vi "Enable SPI Digital Lines(CLIP).vi"(7 "Set?":bool=TRUE, 8 "error in":errorcluster, 9 "Enable":bool[](array[boolean])=[TRUE, FALSE, TRUE, TRUE, TRUE, TRUE, TRUE, TRUE, TRUE], 10 "Enable Lines":T1={"SCLK_en"="sbRIO-9651 Socket\\PMOD1_Pin3_enable", "MISO_en"="sbRIO-9651 Socket\\PMOD1_Pin3_enable", "MOSI_en"="sbRIO-9651 Socket\\PMOD1_Pin3_enable", "CS0_en"="sbRIO-9651 Socket\\PMOD1_Pin3_enable", "CS1_en"="sbRIO-9651 Socket\\PMOD1_Pin3_enable", "CS2_en"="sbRIO-9651 Socket\\PMOD1_Pin3_enable", "CS3_en"="sbRIO-9651 Socket\\PMOD1_Pin3_enable", "CS4_en"="sbRIO-9651 Socket\\PMOD1_Pin3_enable", "CS5_en"="sbRIO-9651 Socket\\PMOD1_Pin3_enable"}, 11 "SPI DIO Lines":T2={"SCLK"="Port0/DIO0", "MISO"="Port0/DIO1", "MOSI"="Port0/DIO2", "CS 0"="Port0/DIO4", "CS 1"="Port0/DIO5", "CS 2"="Port0/DIO6", "CS 3"="Port0/DIO7", "CS 4"="Port0/DIO8", "CS 5"="Port0/DIO9"}) -> (0 "error out":errorcluster, 3 "Chip Select DIO Lines":T2={"SCLK"="Port0/DIO3", "MISO"="Port0/DIO3", "MOSI"="Port0/DIO3", "CS 0"="Port0/DIO4", "CS 1"="Port0/DIO4", "CS 2"="Port0/DIO1", "CS 3"="Port0/DIO4", "CS 4"="Port0/DIO4", "CS 5"="Port0/DIO4"})   [LabVIEW 2014]
uses:
  <vilib>/SPIAPI/DIO/SPI Digital IO Lines.ctl
  <vilib>/SPIAPI/DIO/SPI DIO Enable Lines.ctl
  <vilib>/rvi/eio/common/nirviEmuTemplateMethod_errors.vi
  <vilib>/eio/EIONode/EIONode.xnode
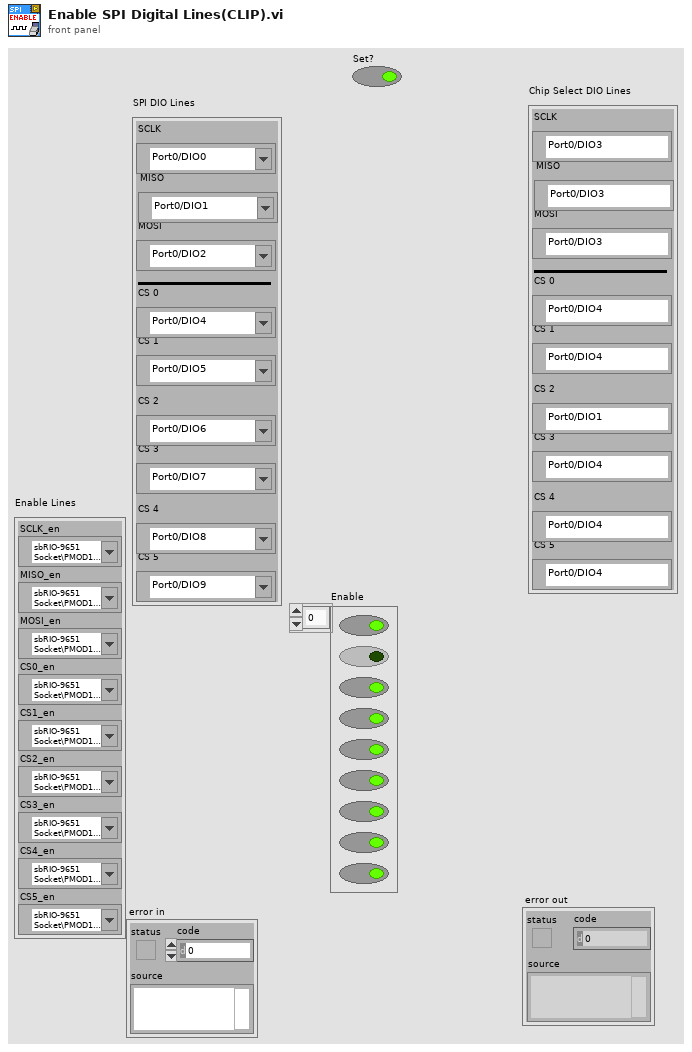
[diagram p1: front panel]
types:
  T1 = typedef "SPI DIO Enable Lines.ctl" = cluster{"SCLK_en":refnum<k21>, "MISO_en":refnum<k21>, "MOSI_en":refnum<k21>, "CS0_en":refnum<k21>, "CS1_en":refnum<k21>, "CS2_en":refnum<k21>, "CS3_en":refnum<k21>, "CS4_en":refnum<k21>, "CS5_en":refnum<k21>}
  T2 = typedef "SPI Digital IO Lines.ctl" = cluster{"SCLK":refnum<k21>, "MISO":refnum<k21>, "MOSI":refnum<k21>, "CS 0":refnum<k21>, "CS 1":refnum<k21>, "CS 2":refnum<k21>, "CS 3":refnum<k21>, "CS 4":refnum<k21>, "CS 5":refnum<k21>}
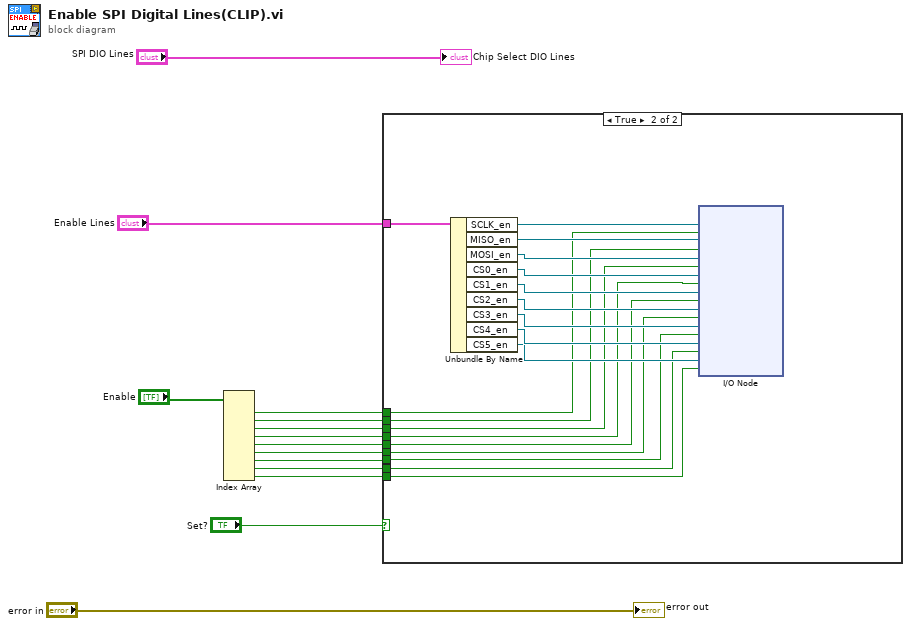
[diagram p0: block diagram]
diagram:
  n1 = Index Array(array="Enable") -> (element #1=w10:bool, element #2=w9:bool, element #3=w8:bool, element #4=w7:bool, element #5=w6:bool, element #6=w5:bool, element #7=w4:bool, element #8=w3:bool, element #9=w2:bool)  [unwired: 9 in]
  n2 = case shown="True" "Set?" {
    tunnel: "Enable Lines" -> [_ w33]
    tunnel: w10 -> [_ w23]
    tunnel: w9 -> [_ w22]
    tunnel: w8 -> [_ w21]
    tunnel: w7 -> [_ w20]
    tunnel: w6 -> [_ w19]
    tunnel: w5 -> [_ w18]
    tunnel: w4 -> [_ w17]
    tunnel: w3 -> [_ w16]
    tunnel: w2 -> [_ w15]
    frame False {
    }
    frame True {
      n3 = Unbundle By Name(w33) -> ("SCLK_en"=w32:refnum<k21>, "MISO_en"=w31:refnum<k21>, "MOSI_en"=w30:refnum<k21>, "CS0_en"=w29:refnum<k21>, "CS1_en"=w28:refnum<k21>, "CS2_en"=w27:refnum<k21>, "CS3_en"=w26:refnum<k21>, "CS4_en"=w25:refnum<k21>, "CS5_en"=w24:refnum<k21>)
      n4 = xnode "I/O Node"("I/O Item"=w23, "FPGA I/O In"=w32, "I/O Item"=w22, "FPGA I/O In"=w31, "I/O Item"=w21, "FPGA I/O In"=w30, "I/O Item"=w20, "FPGA I/O In"=w29, "I/O Item"=w19, "FPGA I/O In"=w28, "I/O Item"=w18, "FPGA I/O In"=w27, "I/O Item"=w17, "FPGA I/O In"=w26, "I/O Item"=w16, "FPGA I/O In"=w25, "I/O Item"=w15, "FPGA I/O In"=w24) -> ()  [unwired: 9 out]
    }
  }
  "Chip Select DIO Lines" <- "SPI DIO Lines"
  "error out" <- "error in"
